vi "Check Servo Messages.vi"(8 "error in (no error)":errorcluster, 10 "queued timestamp":timestamp, 11 "servo queue":refnum<queue>) -> (0 "error out":errorcluster)   [LabVIEW 2020]
uses:
  General Hardware.lvclass
  Actuators/Servos/Servo.lvclass
  C:/Users/jharw/Documents/1 Folder to Rule them All/UMD/Inflation-Apparatus/src/Hardware/Actuators/Actuator.lvclass
  C:/Users/jharw/Documents/1 Folder to Rule them All/UMD/Inflation-Apparatus/src/Hardware/General Hardware.lvclass
  C:/Users/jharw/Documents/1 Folder to Rule them All/UMD/Inflation-Apparatus/src/Hardware/Actuators/Servos/Servo.lvclass
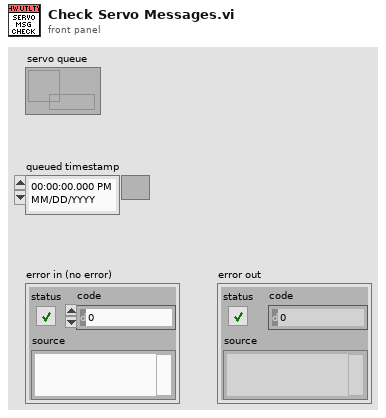
[diagram p1: front panel]
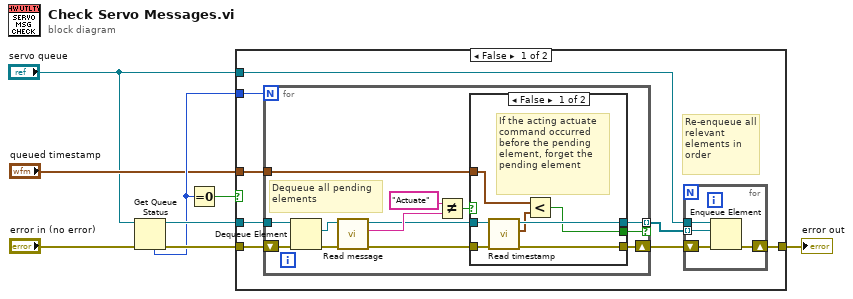
[diagram p0: block diagram]
diagram:
  n1 = Get Queue Status(queue="servo queue", error in (no error)="error in (no error)") -> (queue out=w5:refnum<queue>, error out=w6:errorcluster, # elements in queue=w3:i32)  [unwired: 1 in, 5 out]
  n2 = Equal To 0?(x=w3) -> (x = 0?=w4:bool)
  n3 = case shown="False" w4 {
    tunnel: [w11 w44] -> w8
    tunnel: w6 -> [w16 w44]
    tunnel: w5 -> [w15 _]
    tunnel: w3 -> [w14 _]
    tunnel: "queued timestamp" -> [w13 _]
    tunnel: "servo queue" -> [w10 _]
    frame False {
      # "Re-enqueue all relevant elements in order"
      n4 = for {
        N: w14 -> [_]
        tunnel: w15 -> [w32]
        shift-right: [w24] -> w12
        shift-left: w16 -> [w33]
        tunnel: [w26] -> w9 mode=indexing if=w21
        tunnel: w13 -> [w22]
        # "Dequeue all pending elements"
        n5 = Dequeue Element(queue=w32, error in (no error)=w33) -> (element=w31:refnum<class "Servo.lvclass">, error out=w30:errorcluster)  [unwired: 1 in, 2 out]
        n6 = call "Read message.vi"("error in (no error)"=w30, "General Hardware in"=w31) -> ("error out"=w25:errorcluster, "message"=w29:string, "General Hardware out"=w27:refnum<class "Servo.lvclass">)  [unwired: 7 in]
        n7 = Not Equal?(x="Actuate", y=w29) -> (x != y?=w23:bool)
        n8 = case shown="False" w23 {
          selector: w23 -> [_ w43]
          tunnel: w27 -> [w40 w42]
          tunnel: [w39 w42] -> w26
          tunnel: w25 -> [w38 w41]
          tunnel: [w37 w41] -> w24
          tunnel: w22 -> [w36 _]
          tunnel: [w34 w43] -> w21
          frame False {
            # "If the acting actuate command occurred before the pending element, forget the pending element"
            n9 = call "Read timestamp.vi"("error in (no error)"=w38, "General Hardware in"=w40) -> ("error out"=w37:errorcluster, "timestamp"=w35:timestamp, "General Hardware out"=w39:refnum<class "Servo.lvclass">)  [unwired: 7 in]
            n10 = Less?(x=w36, y=w35) -> (x < y?=w34:bool)
          }
          frame True {
            # "If the pending element is not an actuate command, save the element"
          }
        }
      }
      n11 = for {
        tunnel: w10 -> [w18]
        shift-right: [w19] -> w11
        shift-left: w12 -> [w20]
        tunnel: w9 -> [w17] mode=indexing
        n12 = Enqueue Element(queue=w18, element=w17, error in (no error)=w20) -> (error out=w19:errorcluster)  [unwired: 1 in, 2 out]
      }
    }
    frame True {
      # "If no pending elements, do nothing"
    }
  }
  "error out" <- w8
